vi "Close.vi"(8 "error in":errorcluster, 11 "Color in":refnum<class "Color.lvclass">) -> (0 "error out":errorcluster, 3 "Color out":refnum<class "Color.lvclass">)   [LabVIEW 2024, in "SourceGrid.lvlib" / "Color.lvclass"]
uses:
  Color.lvclass
  Color.lvclass/Color.ctl
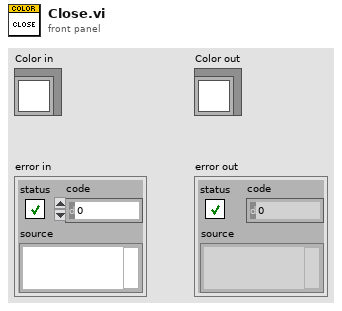
[diagram p1: front panel]
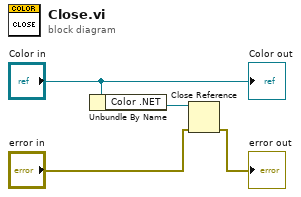
[diagram p0: block diagram]
diagram:
  n1 = Unbundle By Name("Color in") -> ("Color .NET"=w3:refnum<k24>)
  n2 = Close Reference(reference=w3, error in (no error)="error in") -> (error out=→"error out":errorcluster)
  "Color out" <- "Color in"
